vi "Fetch Data DVR.vi"(0 "device session in":refnum<class "Device Session.lvclass">, 1 "timeout (ms)":i32=10000, 5 "number of samples":u32=1000, 11 "error in":errorcluster) -> (4 "device session out":refnum<class "Device Session.lvclass">, 6 "data":refnum<data-value>, 8 "scaling coefficients":cluster{"gain":dbl, "offset":dbl}[](array[cluster]), 10 "samples fetched":u32, 15 "error out":errorcluster)   [LabVIEW 2015, in "Device Session.lvclass"]
doc: "Fetches acquired samples and returns them in a data value reference.\n\n<B>Input Parameters</B>\n\n<B>device session in</B> is a reference to the session containing sessions to all instrument design libraries used in this sample project. This parameter is obtained from the 'Open Session' VI.\n\n<B>number of samples</B> specifies the number of samples per channel to fetch. The default value is 1,000.\n\n<B>timeout (ms)</B> specifies the maximum amount of time to wait for the specified number of samples to be fetched. The default value is 10,000.\n\n<B>error in</B> describes error conditions that occur before this node runs. This input provides standard 'error in' functionality.\n\n<B>Output Parameters</B>\n\n<B>device session out</B> passes a reference to the session to the next VI.\n\n<B>data</B> returns a data value reference with the sample data. You can pass this reference to the 'Deinterleave' VI to obtain a two-dimensional array of deinterleaved samples.\n\n<B>scaling coefficients</B> returns an array of scaling coefficients for each streamed channel, which you can use to convert the returned data to Volts.\n\n<B>samples fetched</B> returns the number of samples per channel fetched.\n\n<B>error out</B> contains error information. This output provides standard 'error out' functionality."
uses:
  Device Session.lvclass
  Device Session.lvclass/Device Session.ctl
  FPGA Refnum.ctl
  <instrlib>/_niInstr/Data Manipulation/v1/Host/Private/Copy to New External Data Value Reference I161D.vi
  <vilib>/rvi/interface/common/dynamic/niFpgaDynamicGetExecutionMode.vi
  <vilib>/Utility/error.llb/Error Cluster From Error Code.vi
  <vilib>/rvi/errors/niLvFpgaAdjustHostInterfaceError.vi
  <instrlib>/_niInstr/Data Manipulation/v1/Host/Private/Map C Error to DataManip Error.vi
  <instrlib>/_niInstr/Data Manipulation/v1/Host/Private/Data Manipulation Error Handler.vi
  <vilib>/rvi/interface/nirviMethod/nirviMethod.xnode
  <vilib>/FPGA/interface/niFpgaViExecutionMode.ctl
  <vilib>/rvi/errors/niLvFpgaMergeErrorWithErrorCode.vi
  <instrlib>/_niInstr/Data Manipulation/v1/Host/niInstr Data Manipulation v1 Host.lvlib
  <vilib>/FPGAPlugInAG/Dynamic/niLvFpga_AcquireReadRegionFifo_Dynamic.vi
  <vilib>/FPGAPlugInAG/Dynamic/niLvFpga_ReadFifo_Dynamic.vi
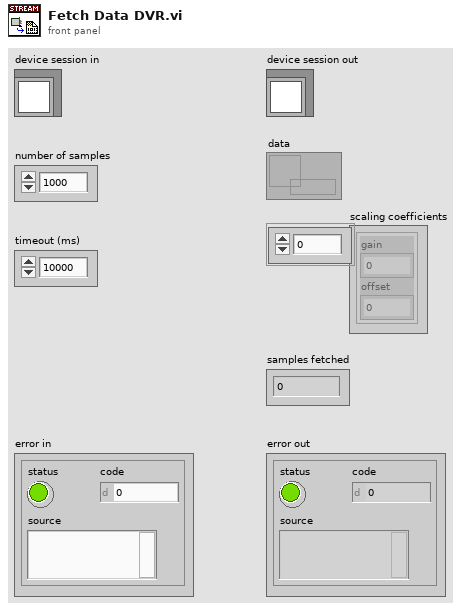
[diagram p1: front panel]
types:
  T1 = typedef "Device Session.lvclass/FPGA Refnum.ctl" = refnum<k20>
  T2 = typedef "Device Session.lvclass/Device Session Object.ctl" = cluster{"ni5171R FPGA Reference":T1, "niHSAI config":refnum<class "niHSAI Config v1 Host.lvclass">, "configured scaling coefficients":cluster{"gain":dbl, "offset":dbl}[], "number of channels to stream":u8, "selected acq channels":bool[], "number of channels":u32, "actual channel configuration":T3[], "configured channels":bool[], "sample clock rate (Hz)":dbl}
  T3 = typedef "niHSAI Types v1 Host.lvlib/Channel Configuration.ctl" = cluster{"channel":u32, "coupling":T4, "impedance":T5, "bandwidth":T6, "vertical range":dbl, "vertical offset":dbl}
  T4 = typedef "niHSAI Types v1 Host.lvlib/Coupling.ctl" = enum8{"Default", "DC", "AC"}
  T5 = typedef "niHSAI Types v1 Host.lvlib/Impedance.ctl" = enum8{"Default", "1 mega ohm", "50 ohm"}
  T6 = typedef "niHSAI Types v1 Host.lvlib/Bandwidth.ctl" = enum8{"Default", "Full Bandwidth", "Anti-alias Filter"}
  T7 = typedef "niFpgaViExecutionMode.ctl" = enum16{"FPGA Target", "Simulation (Simulated I/O)", "Simulation (Real I/O)", "Third-Party Simulation"}
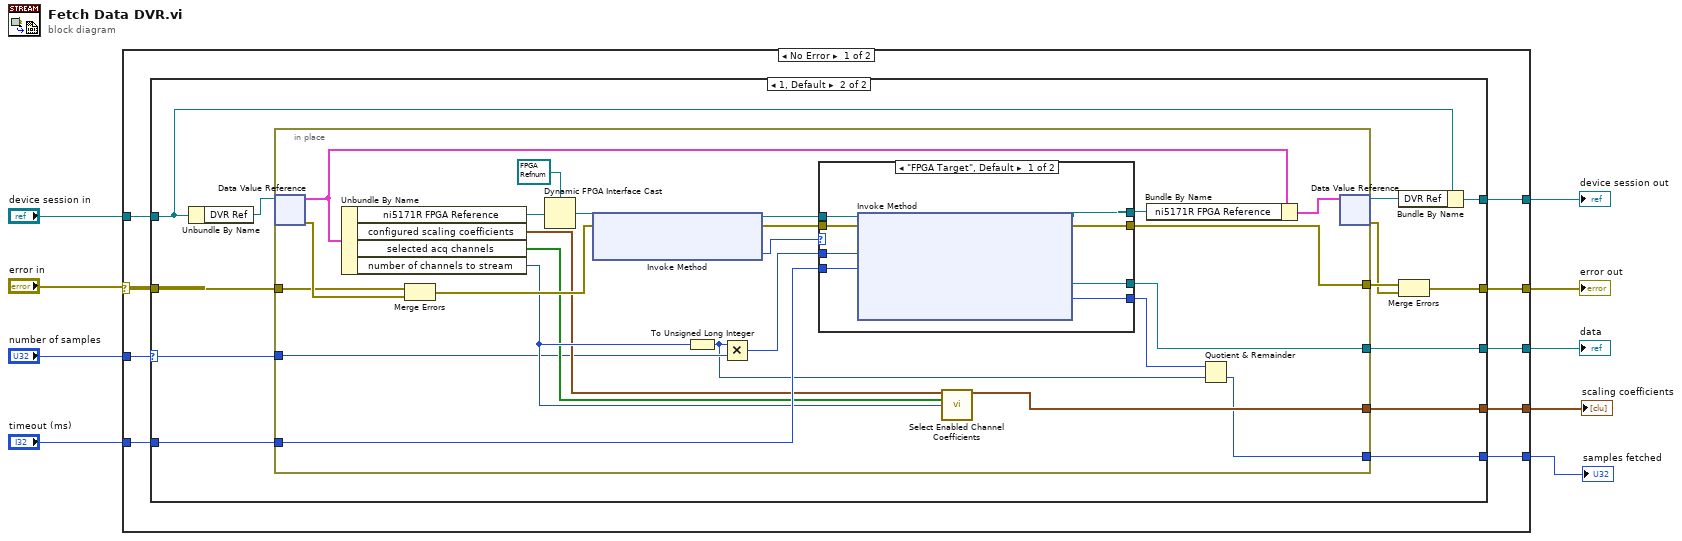
[diagram p0: block diagram]
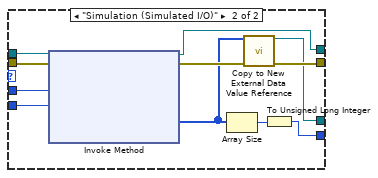
[diagram p3: hidden frame]
diagram:
  n1 = case shown="No Error" "error in" {
    selector: "error in" -> [w18 w78]
    tunnel: [w14 w78] -> w8
    tunnel: "device session in" -> [w16 w77]
    tunnel: [w15 w77] -> w6
    tunnel: "timeout (ms)" -> [w17 _]
    tunnel: [w13 _] -> w3
    tunnel: "number of samples" -> [w12 _]
    tunnel: [w11 _] -> w2
    tunnel: [w10 _] -> w1
    frame No Error {
      n2 = case shown="1, Default" w12 {
        selector: w12 -> [_ w26]
        tunnel: w18 -> [w20 w33]
        tunnel: w17 -> [_ w32]
        tunnel: w16 -> [w19 w29]
        tunnel: [w19 w23] -> w15
        tunnel: [w20 w28] -> w14
        tunnel: [_ w27] -> w13
        tunnel: [_ w22] -> w11
        tunnel: [_ w21] -> w10
        frame 0 {
        }
        frame 1, Default {
          n3 = Unbundle By Name(w29) -> ("DVR Ref"=w31:refnum<data-value>)
          n4 = in-place {
            in-place-border: w33 -> [w54]
            in-place-border: w26 -> [w37]
            in-place-border: w32 -> [w53]
            in-place-border: [w38] -> w25
            in-place-border: [w52] -> w27
            in-place-border: [w39] -> w22
            in-place-border: [w34] -> w21
            n5 = in-place-dvr #1(w31) -> (w57:T2, w55:errorcluster)
            n6 = Unbundle By Name(w57) -> ("ni5171R FPGA Reference"=w45:T1, "configured scaling coefficients"=w40:cluster{"gain":dbl, "offset":dbl}[], "selected acq channels"=w41:bool[], "number of channels to stream"=w42:u8)
            n7 = Merge Errors(w54, w55) -> (w49:errorcluster)
            n8 = Dynamic FPGA Interface Cast(Session In=T1 refnum ("FPGA Interface"), Type=w45) -> (Session Out=w44:T1)
            n9 = xnode "Invoke Method"("FPGA VI Reference In"=w44, "error in"=w49) -> ("FPGA VI Reference Out"=w50:T1, "error out"=w48:errorcluster, "FPGA VI Execution Mode"=w47:T7)
            n10 = To Unsigned Long Integer(number=w42) -> (unsigned 32bit integer=w35:u32)
            n11 = Multiply(x=w35, y=w37) -> (x*y=w43:u32)
            n12 = case shown="\"FPGA Target\", Default" w47 {
              tunnel: [w65 w71] -> w38
              tunnel: w43 -> [w64 w69]
              tunnel: w53 -> [w63 w68]
              tunnel: [w59 w67] -> w52
              tunnel: [w62 w70] -> w51
              tunnel: w50 -> [w61 w75]
              tunnel: w48 -> [w60 w74]
              tunnel: [w58 w66] -> w36
              frame "FPGA Target", Default {
                n13 = xnode "Invoke Method"("FPGA VI Reference In"=w61, "error in"=w60, "Number of Elements"=w64, "Timeout (ms)"=w63) -> ("FPGA VI Reference Out"=w62:T1, "error out"=w65:errorcluster, "Read Region Reference"=w59:refnum<data-value>, "Elements In Region"=w58:u32)  [unwired: 1 out]
              }
              frame "Simulation (Simulated I/O)" {
                n14 = xnode "Invoke Method"("FPGA VI Reference In"=w75, "error in"=w74, "Number of Elements"=w69, "Timeout (ms)"=w68) -> ("FPGA VI Reference Out"=w70:T1, "error out"=w73:errorcluster, "Data"=w72:i16[])  [unwired: 1 out]
                n15 = Array Size(array=w72) -> (size(s)=w76:i32)
                n16 = call-poly <instrlib>:"Copy to New External Data Value Reference.vi"("array"=w72, "error in"=w73) -> ("output array reference"=w67:refnum<data-value>, "error out"=w71:errorcluster)  [unwired: 12 in]
                n17 = To Unsigned Long Integer(number=w76) -> (unsigned 32bit integer=w66:u32)
              }
            }
            n18 = call "Select Enabled Channel Coefficients.vi"("configured scaling coefficients"=w40, "selected acq channels to stream"=w41, "number of selected acq channels to stream"=w42) -> ("streamed scaling coefficients"=w39:cluster{"gain":dbl, "offset":dbl}[])  [unwired: 12 in]
            n19 = Bundle By Name(cluster=w57, "ni5171R FPGA Reference"=w51) -> (w56:T2)
            n20 = Quotient & Remainder(x=w36, y=w35) -> (floor(x/y)=w34:u32)  [unwired: 1 out]
            n21 = in-place-dvr #1(w56) -> (w30:refnum<data-value>, w24:errorcluster)
          }
          n22 = Bundle By Name(cluster=w29, "DVR Ref"=w30) -> (w23:refnum<class "Device Session.lvclass">)
          n23 = Merge Errors(w25, w24) -> (w28:errorcluster)
        }
      }
    }
    frame Error {
    }
  }
  "error out" <- w8
  "device session out" <- w6
  "data" <- w3
  "scaling coefficients" <- w2
  "samples fetched" <- w1
